vi "Log Data to File.vi"() -> ()   [LabVIEW 2017]
panel:
  out "Temperature Data":dbl format="%.1g"
  in  "File Path":path=path "M:/Work/Lab/Lab Work/Master/Industrial IT/OPC Lab/Example Code/data.lvm"
  in  "Record Data":bool
  in  "Stop Button":bool
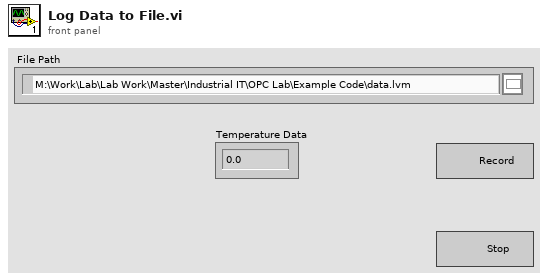
[diagram p1: front panel]
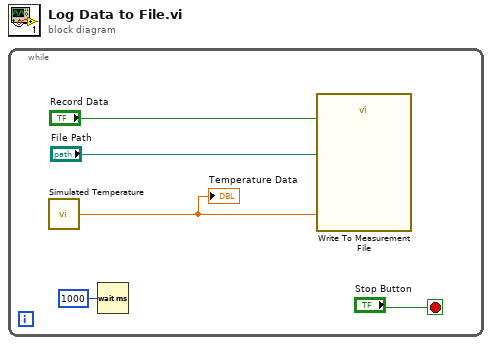
[diagram p0: block diagram]
diagram:
  n1 = while {
    stop <- "Stop Button" stop-if-true
    n2 = call "Simulated Temperature.vi"() -> ("Temperature Value"=w1:dbl)  [unwired: 2 in]
    "Temperature Data" <- w1
    n3 = Wait (ms)(milliseconds to wait=u32 1000) -> ()  [unwired: 1 out]
    n4 = call "Write To Measurement File"("Signals"=w1, "Enable"="Record Data", "Filename"="File Path") -> ()  [unwired: 14 in, 3 out]
  }
